vi "Periodic Tasks.vi"(8 "error in":errorcluster) -> ()   [LabVIEW 2016]
doc: "This VI runs in parallel to other tasks. It can contain as many user-defined periodic loops as you need. These can carry out PID or other sorts of timed response."
uses:
  <vilib>/Rock Robotics/WPI/Utilities/WPI_GetSetVariantRefNum.vi
  Robot Global Data.vi
  <vilib>/Rock Robotics/Network Tables/NT Write Number.vi
  <vilib>/Rock Robotics/Network Tables/NT Write Numeric Array.vi
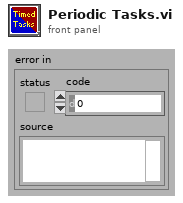
[diagram p1: front panel]
types:
  T1 = typedef "WPI_RobotDriveDevRef.ctl" = cluster{"DevStatus":errorcluster, "Motors[]":T2[], "Square Inputs":bool, "Max Output":dbl}
  T2 = typedef "WPI_MotorControlDeviceRef.ctl" = cluster{"DeviceStatus":errorcluster, "Type":T3, "PWM":cluster{"PWM Channel":T4, "DeadBand":T5}, "CAN":cluster{"Device Number":u8, "SetOutput VI Ref":variant, "GetOutput VI Ref":variant, "Enable VI Ref":variant, "Disable VI Ref":variant, "Data":variant}, "Invert":bool}
  T3 = typedef "WPI_MotorControlType.ctl" = enum16{"PWM", "CAN"}
  T4 = typedef "FPGA_DIOPWMChannel.ctl" = enum8{"PWM 0", "PWM 1", "PWM 2", "PWM 3", "PWM 4", "PWM 5", "PWM 6", "PWM 7", "PWM 8", "PWM 9", "PWM MXP 0", "PWM MXP 1", "PWM MXP 2", "PWM MXP 3", "PWM MXP 4", "PWM MXP 5", "PWM MXP 6", "PWM MXP 7", "PWM MXP 8", "PWM MXP 9", "Invalid"}
  T5 = typedef "WPI_PWMDeadband.ctl" = cluster{"Name":string, "maxPositivePwm":i32, "minPositivePwm":i32, "centerPwm":i32, "maxNegativePwm":i32, "minNegativePwm":i32, "angularRange":u16}
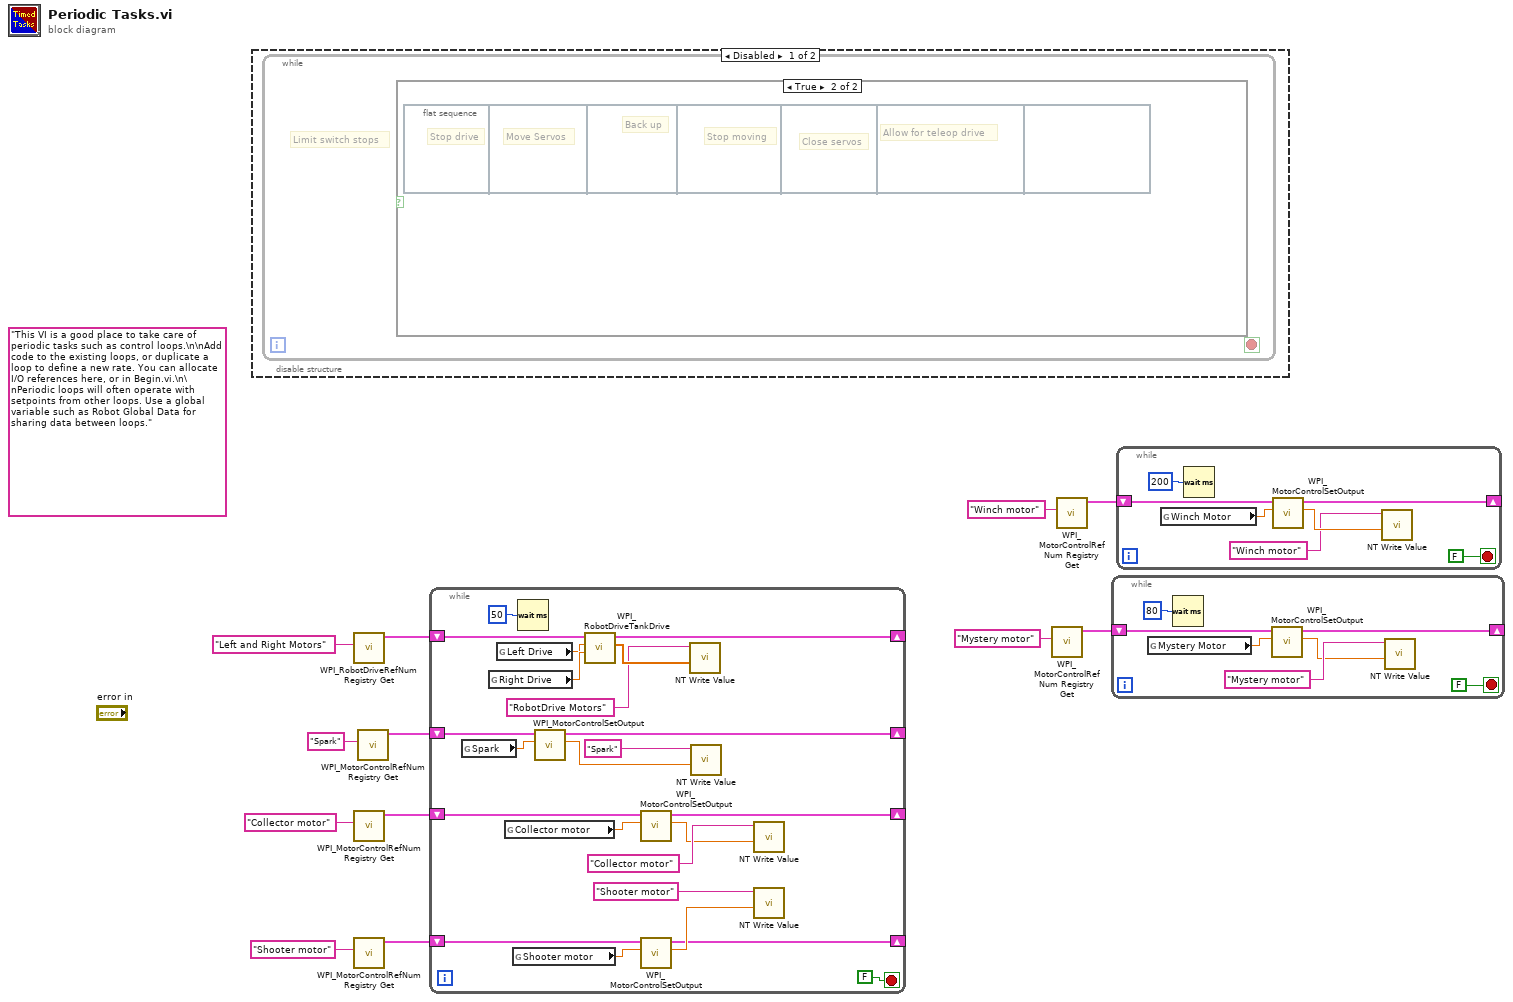
[diagram p0: block diagram]
diagram:
  (unwired) "This VI is a good place to take care of periodic tasks such as control loops.\n\nAdd code to the existing loops, or duplicate a loop to define a new rate. You can allocate I/O references here, or in Begin.vi.\n\nPeriodic loops will often operate with setpoints from other loops. Use a global variable such as Robot Global Data for sharing data between loops."
  n1 = disable-structure shown="Disabled" {
    frame Disabled {
      n2 = while {
        stop <- _ stop-if-true
        # "Limit switch stops"
        n3 = case shown="True" {
          selector: _ -> [_ _]
          frame False {
          }
          frame True {
            n4 = flat-sequence {
              frame #0 {
                # "Stop drive"
              }
              frame #1 {
                # "Move Servos"
              }
              frame #2 {
                # "Back up"
              }
              frame #3 {
                # "Stop moving"
              }
              frame #4 {
                # "Close servos"
              }
              frame #5 {
                # "Allow for teleop drive"
              }
              frame #6 {
              }
            }
          }
        }
      }
    }
    frame Enabled {
    }
  }
  n5 = call <vilib>:"WPI_RobotDriveRefNum Registry Get.vi"("refnum name"="Left and Right Motors") -> ("RobotDriveDevRef"=w11:T1)  [unwired: 1 in, 9 out]
  n6 = call <vilib>:"WPI_MotorControlRefNum Registry Get.vi"("refnum name"="Collector motor") -> ("MotorControlDevRef"=w8:T2)  [unwired: 9 in, 1 out]
  n7 = call <vilib>:"WPI_MotorControlRefNum Registry Get.vi"("refnum name"="Shooter motor") -> ("MotorControlDevRef"=w6:T2)  [unwired: 9 in, 1 out]
  n8 = call <vilib>:"WPI_MotorControlRefNum Registry Get.vi"("refnum name"="Spark") -> ("MotorControlDevRef"=w5:T2)  [unwired: 9 in, 1 out]
  n9 = while {
    shift-right: [w32] -> _
    shift-left: w11 -> [w31]
    shift-right: [w23] -> _
    shift-left: w8 -> [w24]
    shift-right: [w18] -> _
    shift-left: w6 -> [w19]
    shift-right: [w13] -> _
    shift-left: w5 -> [w14]
    stop <- FALSE stop-if-true
    n10 = global read "Robot Global Data.vi" "Spark"() -> (w15:dbl)
    n11 = global read "Robot Global Data.vi" "Right Drive"() -> (w30:dbl)
    n12 = global read "Robot Global Data.vi" "Left Drive"() -> (w29:dbl)
    n13 = global read "Robot Global Data.vi" "Collector motor"() -> (w25:dbl)
    n14 = global read "Robot Global Data.vi" "Shooter motor"() -> (w20:dbl)
    n15 = Wait (ms)(milliseconds to wait=u32 50) -> ()  [unwired: 1 out]
    n16 = call <vilib>:"WPI_MotorControlSetOutput.vi"("Output"=w15, "MotorControlDevRef"=w14) -> ("Motor Output"=w16:dbl, "MotorControlDevRef"=w13:T2)  [unwired: 7 in, 1 out]
    n17 = call <vilib>:"WPI_RobotDriveTankDrive.vi"("Right axis value"=w30, "Left axis value"=w29, "RobotDriveDevRef"=w31) -> ("Motor Values"=w34:dbl[], "RobotDriveDevRef"=w32:T1)  [unwired: 6 in, 1 out]
    n18 = call <vilib>:"WPI_MotorControlSetOutput.vi"("Output"=w25, "MotorControlDevRef"=w24) -> ("Motor Output"=w26:dbl, "MotorControlDevRef"=w23:T2)  [unwired: 7 in, 1 out]
    n19 = call <vilib>:"WPI_MotorControlSetOutput.vi"("Output"=w20, "MotorControlDevRef"=w19) -> ("Motor Output"=w21:dbl, "MotorControlDevRef"=w18:T2)  [unwired: 7 in, 1 out]
    n20 = call-poly <vilib>:"NT Write Value.vi"("Numeric Array"=w34, "Name"="RobotDrive Motors") -> ()  [unwired: 9 in, 1 out]
    n21 = call-poly <vilib>:"NT Write Value.vi"("Numeric"=w16, "Name"="Spark") -> ()  [unwired: 9 in, 1 out]
    n22 = call-poly <vilib>:"NT Write Value.vi"("Numeric"=w26, "Name"="Collector motor") -> ()  [unwired: 9 in, 1 out]
    n23 = call-poly <vilib>:"NT Write Value.vi"("Numeric"=w21, "Name"="Shooter motor") -> ()  [unwired: 9 in, 1 out]
  }
  n24 = call <vilib>:"WPI_MotorControlRefNum Registry Get.vi"("refnum name"="Mystery motor") -> ("MotorControlDevRef"=w1:T2)  [unwired: 9 in, 1 out]
  n25 = call <vilib>:"WPI_MotorControlRefNum Registry Get.vi"("refnum name"="Winch motor") -> ("MotorControlDevRef"=w3:T2)  [unwired: 9 in, 1 out]
  n26 = while {
    shift-right: [w37] -> _
    shift-left: w1 -> [w38]
    stop <- FALSE stop-if-true
    n27 = global read "Robot Global Data.vi" "Mystery Motor"() -> (w39:dbl)
    n28 = Wait (ms)(milliseconds to wait=u32 80) -> ()  [unwired: 1 out]
    n29 = call <vilib>:"WPI_MotorControlSetOutput.vi"("Output"=w39, "MotorControlDevRef"=w38) -> ("Motor Output"=w40:dbl, "MotorControlDevRef"=w37:T2)  [unwired: 7 in, 1 out]
    n30 = call-poly <vilib>:"NT Write Value.vi"("Numeric"=w40, "Name"="Mystery motor") -> ()  [unwired: 9 in, 1 out]
  }
  n31 = while {
    shift-right: [w46] -> _
    shift-left: w3 -> [w47]
    stop <- FALSE stop-if-true
    n32 = global read "Robot Global Data.vi" "Winch Motor"() -> (w48:dbl)
    n33 = Wait (ms)(milliseconds to wait=u32 200) -> ()  [unwired: 1 out]
    n34 = call <vilib>:"WPI_MotorControlSetOutput.vi"("Output"=w48, "MotorControlDevRef"=w47) -> ("Motor Output"=w49:dbl, "MotorControlDevRef"=w46:T2)  [unwired: 7 in, 1 out]
    n35 = call-poly <vilib>:"NT Write Value.vi"("Numeric"=w49, "Name"="Winch motor") -> ()  [unwired: 9 in, 1 out]
  }
